vi "robotoutputs.vi"() -> ()   [LabVIEW 2020]
doc: "This global variable contains current robot state information and actuator setpoints."
panel:
  out "Shooter_Ready":bool
  out "Shooter_Spinning":bool
  out "Selected_Shooter_Setpoint_Angle":dbl
  out "Selected_Shooter_Setpoint_Ratio":dbl
  out "Selected_Shooter_Setpoint_Speed":dbl
  out "Shooter_Upper_Speed_Ratio":dbl
  out "Shooter_Speed_Goal":dbl
  out "Disallowed_Shooter_States":bool[](array[boolean])
  out "Confirmed_Shooter_States":bool[](array[boolean])
  out "Cowl_Goal_Angle":dbl
  out "Turret_Command":dbl
  out "LimeLight_Pipeline_Commanded":T1(ring)
  out "Current_Driver_Profile_Setpoints":dbl[](array[numeric])
  out "LED_Colors":u32[](array[colorbox])
  out "LimeLight_LED_Mode":enum16{"Pipeline Setting", "Off", "Blink", "On"}(ring)=enum."Off"
  out "Force_Low_Gear":bool
  out "Swerve_2_High_Gear_Requested":bool
  out "Swerve_1_High_Gear_Requested":bool
  out "Swerve_3_High_Gear_Requested":bool
  out "Swerve_0_High_Gear_Requested":bool
  out "Swerve_2_Drive_Flip":bool
  out "Swerve_1_Drive_Flip":bool
  out "Swerve_3_Drive_Flip":bool
  out "Swerve_0_Drive_Flip":bool
  out "Swerve_3_Azimuth_Goal (deg)":dbl
  out "Swerve_1_Azimuth_Goal (deg)":dbl
  out "Swerve_2_Azimuth_Goal (deg)":dbl
  out "Swerve_0_Azimuth_Goal (deg)":dbl
  out "Diverting_Power_LEDS":bool
  out "Swerve_Rotation_Command":dbl
  out "Disallowed_Master_States":bool[](array[boolean])
  out "Drive_Mode":enum16{"Driver Control", "Lock Heading"}(ring)
  out "Diverting_Power_Compressor":bool
  out "Field_Oriented":bool
  out "Confirmed_Master_States":bool[](array[boolean])
  out "Boost_Drive_Current_Limit":bool
  out "Swerve_3_Azimuth_Error (deg)":dbl
  out "Swerve_1_Azimuth_Error (deg)":dbl
  out "Swerve_2_Azimuth_Error (deg)":dbl
  out "Swerve_0_Azimuth_Error (deg)":dbl
  out "Swerve_3_Drive_Command":dbl
  out "Swerve_1_Drive_Command":dbl
  out "Swerve_2_Drive_Command":dbl
  out "Swerve_0_Drive_Command":dbl
  # "--master state controller--"
  # "--drivebase subsystem--"
  # "--ball handling subsystem--"
  # "--power management--"
  # "--LL control--"
  # "--LEDs--"
  # "--climber subsystem--"
  # "--shooter subsystem--"
  # "--turret subsystem--"
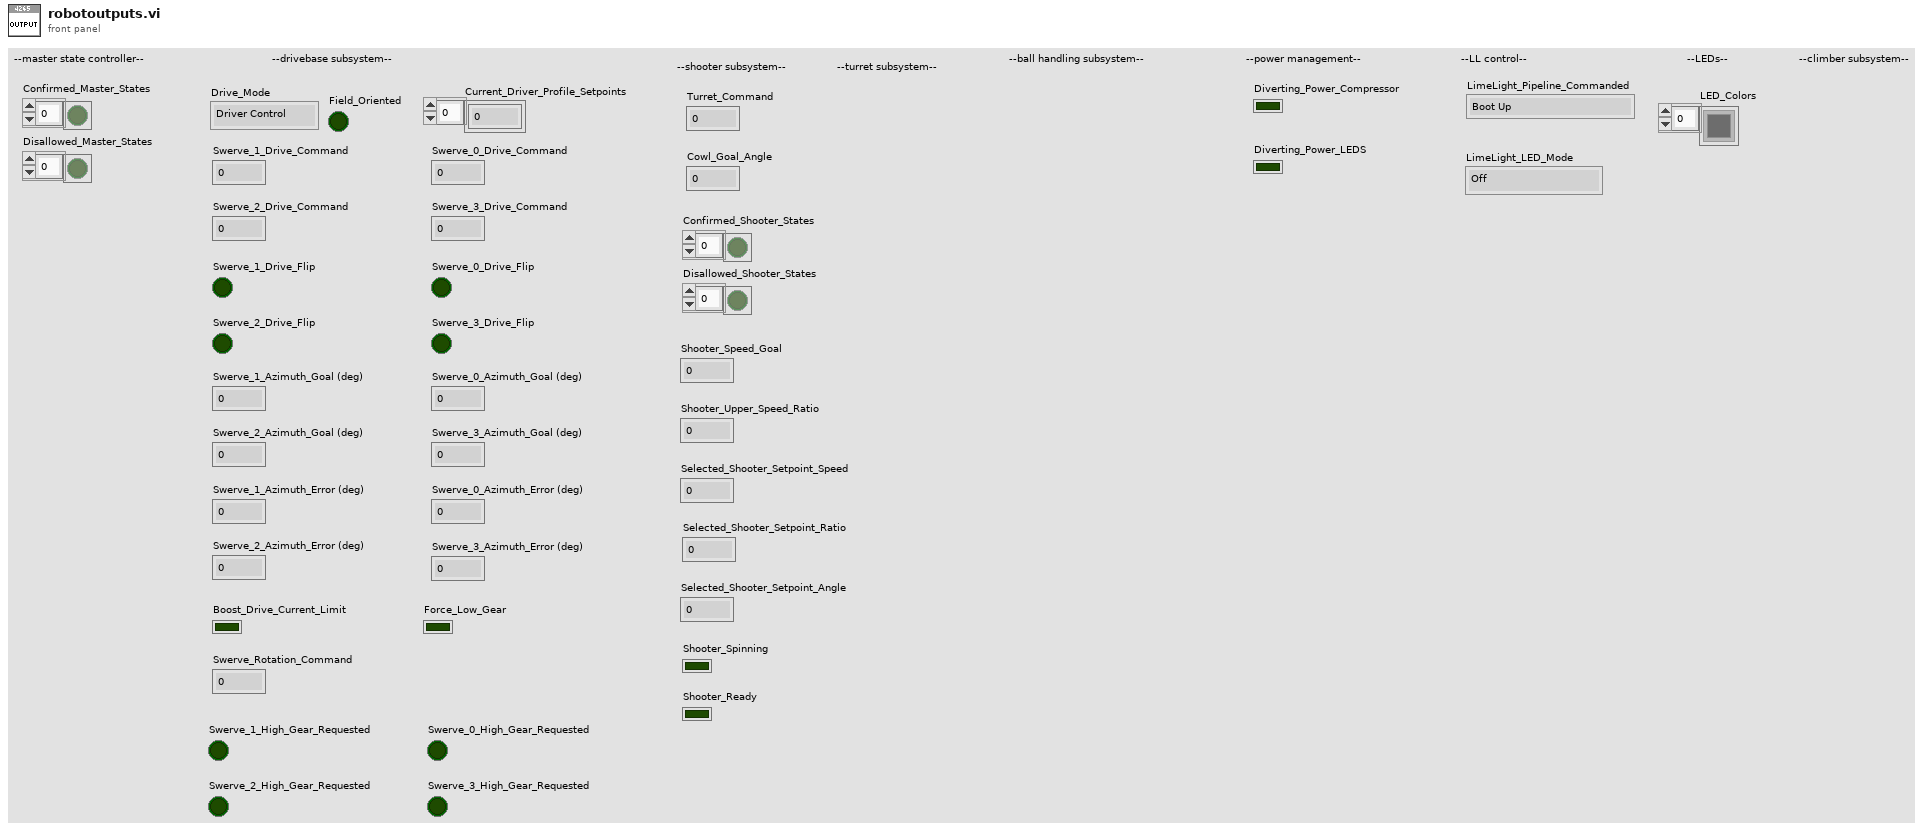
[diagram p1: front panel]
types:
  T1 = enum16{"Boot Up", "Camera Override", "HUB Targeting", "CARGO Tracking"}
diagram:
